vi "Position_Label.vi"(1 "Analysis Info cluster":T1[](array[typedef]) {"Sd Error in Variance" format="%.2f"; "Skew_u" format="%.2f"; "% u'/U" format="%.2f"; "Sd Error in Mean" format="%.2f"; "Kurt_u" format="%.2f"; "u^4" format="%.2f"; "u^3" format="%.2f"; "U" format="%.2f"; "u^2" format="%.2f"}) -> (0 "Position Label":string[](array[string]))   [LabVIEW 2012]
uses:
  Controls/Analysis_info_cluster.ctl
  Controls/Inst_type.ctl
  Controls/Instrument_Array.ctl
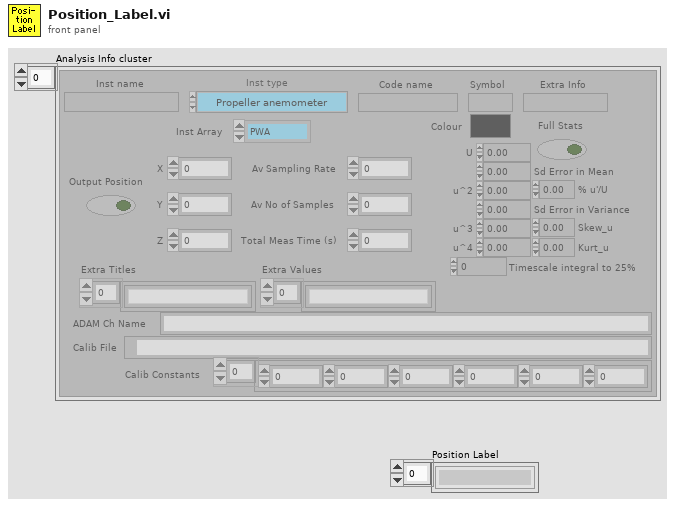
[diagram p1: front panel]
types:
  T1 = typedef "Analysis_info_cluster.ctl" = cluster{"Colour":u32, "Inst type":T2, "Inst name":string, "Symbol":string, "Code name":string, "Extra Info":string, "Inst Array":T3, "Extra Titles":string[], "Extra Values":string[], "U":dbl, "u^2":dbl, "u^3":dbl, "u^4":dbl, "Skew_u":dbl, "Kurt_u":dbl, "Sd Error in Mean":dbl, "% u'/U":dbl, "X":dbl, "Y":dbl, "Z":dbl, "Timescale integral to 25%":dbl, "Sd Error in Variance":dbl, "Calib File":path, "Calib Constants":dbl[], "Output Position":bool, "Full Stats":bool, "Av Sampling Rate":dbl, "Av No of Samples":dbl, "Total Meas Time (s)":dbl, "ADAM Ch Name":string}
  T2 = typedef "Inst_type.ctl" = enum16{"Propeller anemometer", "Raw voltage", "Pressure Transducer", "Pitot-static tube", "Preston tube", "Hot wire", "Cross wire 1", "Cross wire 2", "Generic Linear", "Generic Polynomial", "Generic BackPoly", "Fast FID", "Thermocouple", "Cold wire", "Pulsed Wire", "LDA Vel", "LDA Tran time", "LDA Arr time"}
  T3 = typedef "Instrument_Array.ctl" = enum16{"PWA", "LDA", "Analogue"}
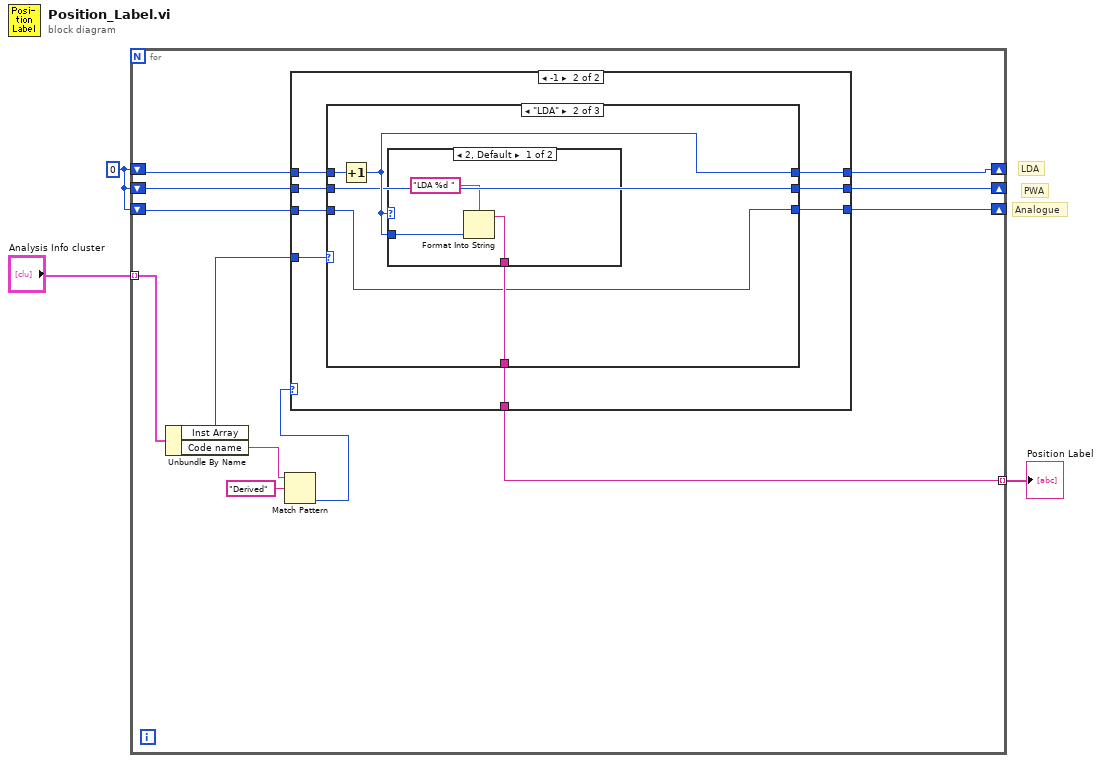
[diagram p0: block diagram]
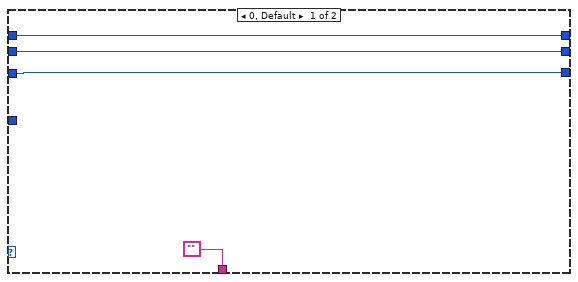
[diagram p2: hidden frame]
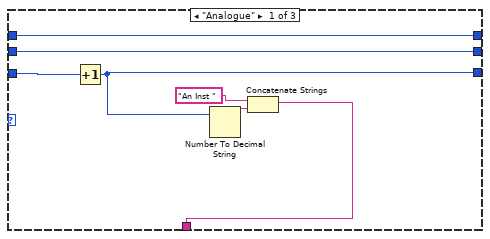
[diagram p3: hidden frame]
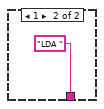
[diagram p4: hidden frame]
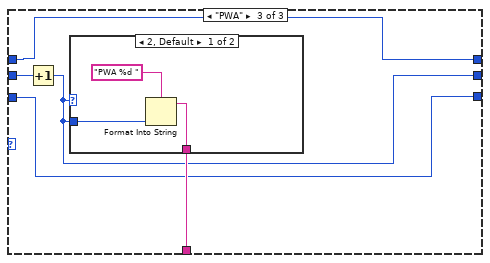
[diagram p5: hidden frame]
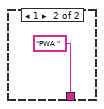
[diagram p6: hidden frame]
diagram:
  w3 = 0
  # "Analogue"
  # "PWA"
  # "LDA"
  n1 = for {
    tunnel: "Analysis Info cluster" -> [w15] mode=indexing
    shift-right: [w8] -> _
    shift-left: w3 -> [w13]
    shift-right: [w7] -> _
    shift-left: w3 -> [w6]
    shift-right: [w5] -> _
    shift-left: w3 -> [w12]
    tunnel: [w4] -> w1 mode=indexing
    n2 = Unbundle By Name(w15) -> ("Inst Array"=w14:T3, "Code name"=w11:string)
    n3 = Match Pattern(string=w11, regular expression="Derived") -> (offset past match=w9:i32)  [unwired: 1 in, 3 out]
    n4 = case shown="-1" w9 {
      tunnel: w14 -> [_ w27]
      tunnel: w13 -> [w19 w26]
      tunnel: w12 -> [w17 w25]
      tunnel: [w19 w24] -> w8
      tunnel: [w18 w23] -> w7
      tunnel: w6 -> [w18 w22]
      tunnel: [w17 w21] -> w5
      tunnel: ["" w20] -> w4
      frame 0, Default {
      }
      frame -1 {
        n5 = case shown="\"LDA\"" w27 {
          tunnel: w26 -> [w28 w39 w44]
          tunnel: [w31 w38 w48] -> w20
          tunnel: w25 -> [w32 w35 w47]
          tunnel: [w28 w37 w44] -> w24
          tunnel: [w29 w36 w45] -> w23
          tunnel: w22 -> [w29 w36 w46]
          tunnel: [w30 w35 w47] -> w21
          frame "Analogue" {
            n6 = Increment(x=w32) -> (x+1=w30:i32)
            n7 = Number To Decimal String(number=w30) -> (decimal integer string=w34:string)  [unwired: 1 out]
            n8 = Concatenate Strings("An Inst ", w34) -> (w31:string)
          }
          frame "LDA" {
            n9 = Increment(x=w39) -> (x+1=w37:i32)
            n10 = case shown="2, Default" w37 {
              tunnel: [w40 "LDA "] -> w38
              tunnel: w37 -> [w42 _]
              frame 2, Default {
                n11 = Format Into String(format string="LDA %d ", w42) -> (resulting string=w40:string)  [unwired: 2 in, 1 out]
              }
              frame 1 {
              }
            }
          }
          frame "PWA" {
            n12 = Increment(x=w46) -> (x+1=w45:i32)
            n13 = case shown="2, Default" w45 {
              tunnel: [w49 "PWA "] -> w48
              tunnel: w45 -> [w51 _]
              frame 2, Default {
                n14 = Format Into String(format string="PWA %d ", w51) -> (resulting string=w49:string)  [unwired: 2 in, 1 out]
              }
              frame 1 {
              }
            }
          }
        }
      }
    }
  }
  "Position Label" <- w1
